vi "Property Node Read Core.vi"(8 "error in (no error)":errorcluster, 10 "property":string, 11 "SLSC Remote in":refnum<class "SLSC Remote.lvclass">) -> (0 "error out":errorcluster, 2 "value":variant, 3 "SLSC Remote out":refnum<class "SLSC Remote.lvclass">)   [LabVIEW 2015, in "SLSC Remote.lvclass"]
uses:
  SLSC Remote.lvclass
  <vilib>/NI/i3 JSON/JSON Generation/Create Value Files/Create Value - Object.vi
  <vilib>/NI/i3 JSON/JSON Generation/Add Object Parameter Files/Add Object Parameter - String.vi
  <vilib>/NI/NI JSONRPC Server Framework/Classes/Server/Format Client Request (Auto-Increment).vi
  <vilib>/httpClient/POSTBuffer.vi
  <vilib>/NI/i3 JSON/JSON Parsing/Get Object Parameter Files/Get Object Parameter - Known Type.vi
  <vilib>/NI/NI JSONRPC Server Framework/Classes/Server/JSONRPC Server.lvclass
  <vilib>/NI/i3 JSON/i3-json.lvlib
  <vilib>/httpClient/LabVIEWHTTPClient.lvlib
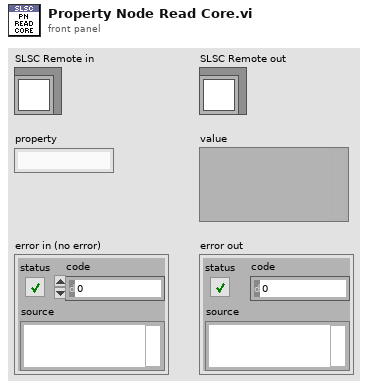
[diagram p1: front panel]
types:
  T1 = typedef "LabVIEWHTTPClient.lvlib/ClientHandle.ctl" = refnum<k1>
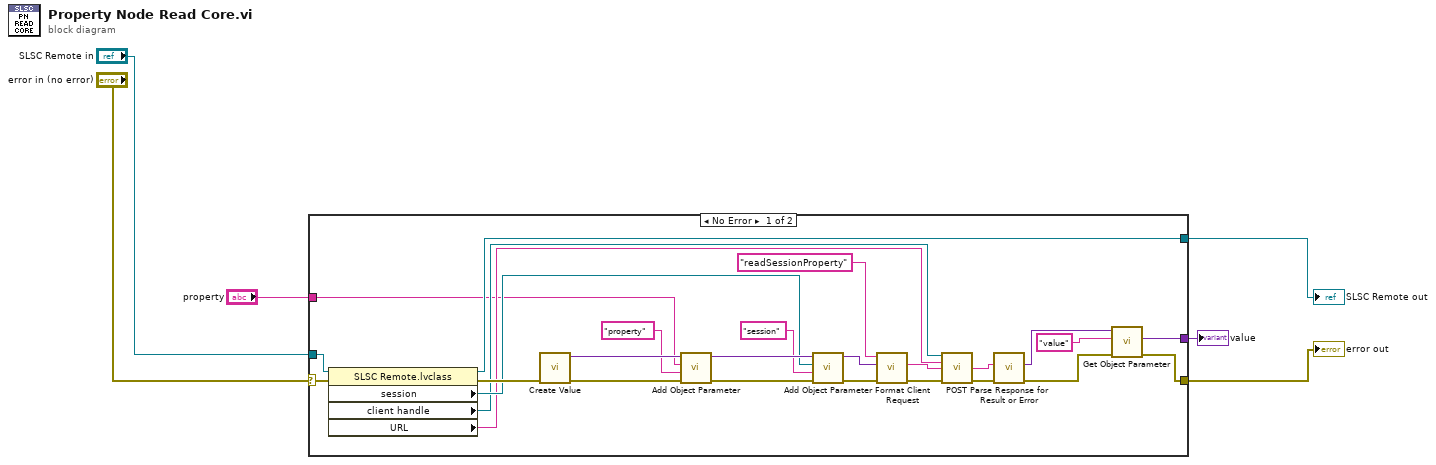
[diagram p0: block diagram]
diagram:
  n1 = case shown="No Error" "error in (no error)" {
    selector: "error in (no error)" -> [w28 w33]
    tunnel: "SLSC Remote in" -> [w31 w34]
    tunnel: [w30 w34] -> w2
    tunnel: [w8 w33] -> w3
    tunnel: [w10 _] -> w6
    tunnel: "property" -> [w7 _]
    frame No Error {
      n2 = property class="SLSC Remote.lvclass"(reference=w31, error in=w28) -> (reference out=w30:refnum<class "SLSC Remote.lvclass">, error out=w27:errorcluster, "session"=w21:refnum<k21>, "client handle"=w17:T1, "URL"=w16:string)
      n3 = call-poly <vilib>:"Create Value.vi"("error in (no error)"=w27) -> ("error out"=w26:errorcluster, "JSON Tree"=w32:variant)  [unwired: 9 in]
      n4 = call-poly <vilib>:"Add Object Parameter.vi"("error in (no error)"=w26, "Name"="property", "String"=w7, "JSON Tree in (JSON Object)"=w32) -> ("error out"=w22:errorcluster, "JSON Tree out (JSON Object)"=w23:variant)  [unwired: 6 in]
      n5 = call-poly <vilib>:"Add Object Parameter.vi"("error in (no error)"=w22, "Name"="session", "String"=w21, "JSON Tree in (JSON Object)"=w23) -> ("error out"=w18:errorcluster, "JSON Tree out (JSON Object)"=w19:variant)  [unwired: 6 in]
      n6 = call-poly <vilib>:"Format Client Request.vi"("error in (no error)"=w18, "params"=w19, "method"="readSessionProperty") -> ("error out"=w15:errorcluster, "Request String"=w24:string)  [unwired: 7 in]
      n7 = call-poly <vilib>:"POST.vi"("client handle"=w17, "url"=w16, "buffer"=w24, "error in (no error)"=w15) -> ("body"=w14:string, "error out"=w13:errorcluster)  [unwired: 8 in, 2 out]
      n8 = call <vilib>:"Parse Response for Result or Error.vi"("error in"=w13, "Response String In"=w14) -> ("error out"=w9:errorcluster, "Result or Error Data"=w11:variant)  [unwired: 7 in, 1 out]
      n9 = call-poly <vilib>:"Get Object Parameter.vi"("error in (no error)"=w9, "Parameter Name"="value", "JSON Tree In (JSON Object)"=w11) -> ("error out"=w8:errorcluster, "Value"=w10:variant)  [unwired: 3 in, 4 out]
    }
    frame Error {
    }
  }
  "value" <- w6
  "error out" <- w3
  "SLSC Remote out" <- w2
